vi "Create.vi"(7 "options":T1, 8 "error in (no error)":errorcluster, 10 "Public Threads":refnum<class "Thread.lvclass">[](array[class]), 11 "Private Threads":refnum<class "Thread.lvclass">[](array[class])) -> (0 "error out":errorcluster, 3 "Thread Manager":refnum<class "Thread Manager.lvclass">)   [LabVIEW 2017, in "DSF Core.lvlib" / "Thread Manager.lvclass"]
uses:
  Thread Manager.lvclass
  Thread/Thread.lvclass
  Thread/DSF Thread Options.ctl
  Thread Manager.lvclass/Thread Manager.ctl
  DSF Core.lvlib
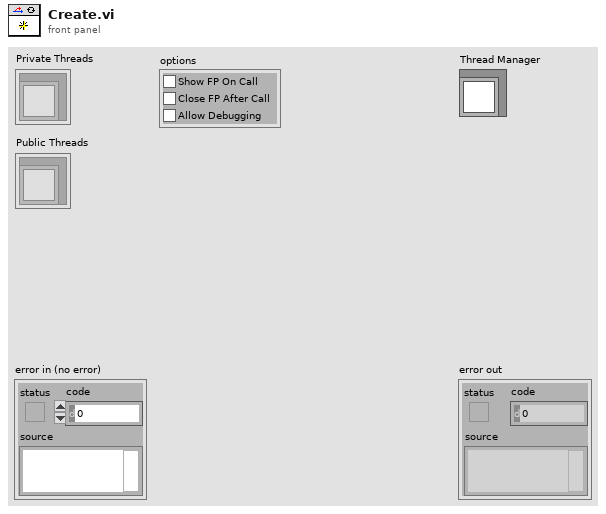
[diagram p1: front panel]
types:
  T1 = typedef "DSF Core.lvlib/DSF Thread Options.ctl" = cluster{"Show FP On Call":bool, "Close FP After Call":bool, "Allow Debugging":bool}
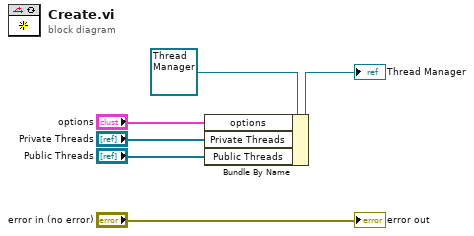
[diagram p0: block diagram]
diagram:
  n1 = Bundle By Name(cluster=refnum<class "Thread Manager.lvclass"> refnum ("Thread Manager in"), "options"="options", "Private Threads"="Private Threads", "Public Threads"="Public Threads") -> (→"Thread Manager":refnum<class "Thread Manager.lvclass">)
  "error out" <- "error in (no error)"
